vi "Async Cleanup.vi"(8 "error in (no error)":errorcluster, 11 "Variables":T1={"Process Ref"=refnum, "Comm Ref"=refnum, "Bus Info"={"Name"="", "Overrides?"=FALSE, "XNET Refs"={"Incoming"="", "Outgoing"=""}, "Port Info"={"Port"="", "Baud Rate"=0, "Termination"=0, "CAN I/O Mode"=0, "FD Baud Rate"=500000, "Priority"=100, "FD ISO Mode"=0}, "Frames"=variant(cluster{"Convert Session":refnum<k21>, "ID":u32, "Length":i32, "Offset":i32}[] [])}, "Stream Refs"={"Addon"="", "Port"="", "Filter Ref"=refnum, "Default Filter"={"ID Filters"=[], "Direction Filter"=enum."Tx/Rx", "Type Filter"=enum."All"}, "Port Settings"={"Mode"=0, "Baud Rate"=0, "Termination"=0, "FD ISO Mode"=0, "FD Baud Rate"=0}}, "Data Refs"={"Port.Status"=refnum, "Frame.Enable"=refnum, "Frame.Signals"=refnum, "Frame.Overrides"=refnum, "Port.Enable"=refnum}} {"Stream Refs"."Port Settings"."FD ISO Mode" items=["ISO", "Non ISO", "ISO Legacy"]; "Stream Refs"."Port Settings"."Termination" items=["Off", "On"]; "Stream Refs"."Port Settings"."Mode" items=["CAN 2.0", "CAN FD", "CAN FD+BRS"]; "Bus Info"."Port Info"."FD ISO Mode" items=["ISO", "Non ISO", "ISO Legacy"]; "Bus Info"."Port Info"."CAN I/O Mode" items=["CAN 2.0", "CAN FD", "CAN FD+BRS"]; "Bus Info"."Port Info"."Termination" items=["Off", "On"]}) -> (0 "error out":errorcluster)   [LabVIEW 2019, in "Ghost Bus Addon Engine.lvlib"]
uses:
  Ghost Bus Addon Engine.lvlib
  Types/RT Async Engine Variables.ctl
  <vilib>/NI/NIVS Inline Async API/_VS Inline Async API/Process/Process.lvclass
  <vilib>/NI/NI VeriStand Addon Network Comm/Engine/VeriStand Comm.lvclass
  Types/RT Bus Settings.ctl
  Types/RT XNET Refs.ctl
  Addon Shared/Types/XNET Port Settings.ctl
  SubModules/CAN-Streaming-Support/Source/Addon/Addon Engine/Types/Engine Stream Refs.ctl
  SubModules/CAN-Streaming-Support/Source/Addon/Addon Shared/Types/Direction Filter.ctl
  SubModules/CAN-Streaming-Support/Source/Addon/Addon Shared/Types/Type Filter.ctl
  SubModules/CAN-Streaming-Support/Source/Addon/Addon Shared/Types/Filter Parameters.ctl
  SubModules/CAN-Streaming-Support/Source/Addon/Addon Engine/Types/Engine Stream Port Settings.ctl
  Types/RT Data Refs.ctl
  <vilib>/NI/NIVS Inline Async API/_Data Access Engine/Data Access Engine/Types/Write.DVR.ctl
  <vilib>/NI/NIVS Inline Async API/_Data Access Engine/Access Type Classes/Write/Write.lvclass
  <vilib>/NI/NIVS Inline Async API/_Data Access Engine/Data Access Engine/Types/Read.DVR.ctl
  <vilib>/NI/NIVS Inline Async API/_Data Access Engine/Access Type Classes/Read/Read.lvclass
  Types/RT Frame Settings.ctl
  <vilib>/Utility/SystemLogging/Write to System Log.vi
  SubModules/CAN-Streaming-Support/Source/Addon/Addon Shared/CAN Stream Support Shared.lvlib
  SubModules/CAN-Streaming-Support/Source/Addon/Addon Engine/CAN Stream Support Engine.lvlib
  <vilib>/NI/NIVS Inline Async API/_Data Access Engine/Data Access Engine/Data Access Engine.lvclass
  Addon Shared/Ghost Bus Addon Shared.lvlib
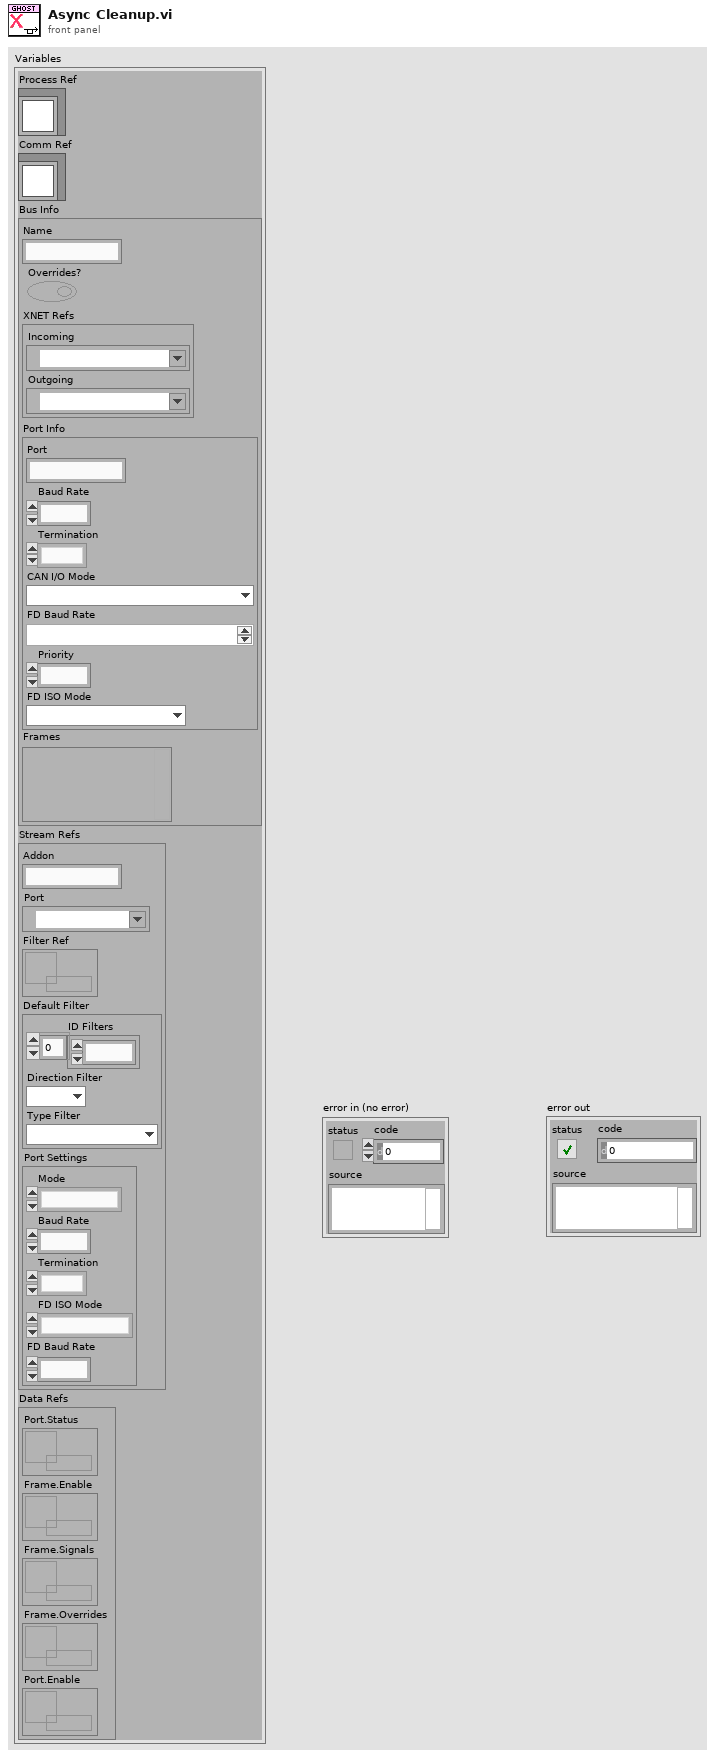
[diagram p1: front panel]
types:
  T1 = typedef "Ghost Bus Addon Engine.lvlib/RT Async Engine Variables.ctl" = cluster{"Process Ref":refnum<class "Process.lvclass">, "Comm Ref":refnum<class "VeriStand Comm.lvclass">, "Bus Info":T2, "Stream Refs":T5, "Data Refs":T10}
  T2 = typedef "RT Bus Settings.ctl" = cluster{"Name":string, "Overrides?":bool, "XNET Refs":T3, "Port Info":T4, "Frames":variant}
  T3 = typedef "Ghost Bus Addon Engine.lvlib/RT XNET Refs.ctl" = cluster{"Incoming":refnum<k21>, "Outgoing":refnum<k21>}
  T4 = typedef "Ghost Bus Addon Shared.lvlib/XNET Port Settings.ctl" = cluster{"Port":string, "Baud Rate":u64, "Termination":u32, "CAN I/O Mode":u32, "FD Baud Rate":u64, "Priority":i32, "FD ISO Mode":u32}
  T5 = typedef "CAN Stream Support Engine.lvlib/Engine Stream Refs.ctl" = cluster{"Addon":string, "Port":refnum<k21>, "Filter Ref":refnum<data-value>, "Default Filter":T6, "Port Settings":T9}
  T6 = typedef "CAN Stream Support Shared.lvlib/Filter Parameters.ctl" = cluster{"ID Filters":u32[], "Direction Filter":T7, "Type Filter":T8}
  T7 = typedef "CAN Stream Support Shared.lvlib/Direction Filter.ctl" = enum16{"Tx/Rx", "Rx", "Tx"}
  T8 = typedef "CAN Stream Support Shared.lvlib/Type Filter.ctl" = enum16{"All", "CAN Data", "CAN Remote", "CAN Bus Error", "CAN 2.0 Data", "CAN FD Data", "CAN FD+BRS Data", "J1939 Data", "Delay", "Log Trigger", "Start Trigger"}
  T9 = typedef "CAN Stream Support Engine.lvlib/Engine Stream Port Settings.ctl" = cluster{"Mode":u32, "Baud Rate":u64, "Termination":u32, "FD ISO Mode":u32, "FD Baud Rate":u64}
  T10 = typedef "Ghost Bus Addon Engine.lvlib/RT Data Refs.ctl" = cluster{"Port.Status":T11, "Frame.Enable":T12, "Frame.Signals":T12, "Frame.Overrides":T12, "Port.Enable":T12}
  T11 = typedef "Data Access Engine.lvlib/Data Access Engine.lvclass/Write.DVR.ctl" = refnum<data-value>
  T12 = typedef "Data Access Engine.lvlib/Data Access Engine.lvclass/Read.DVR.ctl" = refnum<data-value>
  T13 = typedef "Ghost Bus Addon Engine.lvlib/RT Frame Settings.ctl" = cluster{"Convert Session":refnum<k21>, "Length":i32, "Offset":i32, "Enable Offset":i32}
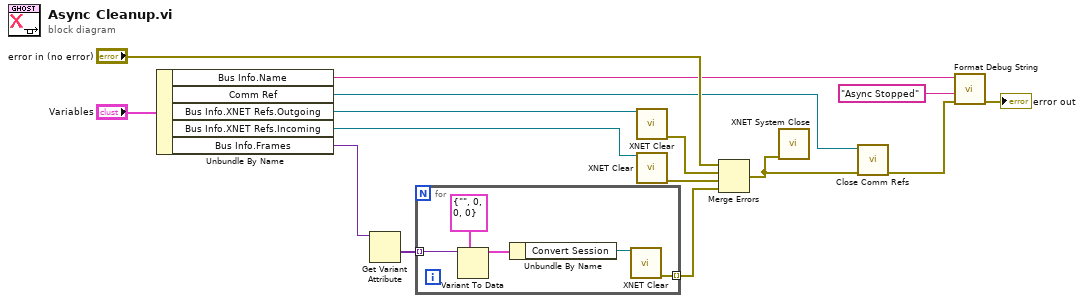
[diagram p0: block diagram]
diagram:
  n1 = Unbundle By Name("Variables") -> ("Bus Info.Name"=w8:string, "Comm Ref"=w3:refnum<class "VeriStand Comm.lvclass">, "Bus Info.XNET Refs.Outgoing"=w15:refnum<k21>, "Bus Info.XNET Refs.Incoming"=w6:refnum<k21>, "Bus Info.Frames"=w2:variant)
  n2 = Get Variant Attribute(Variant=w2) -> (values=w1:variant[])  [unwired: 3 in, 3 out]
  n3 = for {
    tunnel: [w19] -> w4 mode=indexing
    tunnel: w1 -> [w18] mode=indexing
    n4 = Variant To Data(type=T13 {"Convert Session"="", "Length"=0, "Offset"=0, "Enable Offset"=0} ("cluster"), Variant=w18) -> (data=w16:T13)  [unwired: 1 in, 1 out]
    n5 = Unbundle By Name(w16) -> ("Convert Session"=w20:refnum<k21>)
    n6 = call <vilib>:"XNET Clear.vi"("session in"=w20) -> ("error out"=w19:errorcluster)  [unwired: 14 in]
  }
  n7 = call <vilib>:"XNET Clear.vi"("session in"=w15) -> ("error out"=w14:errorcluster)  [unwired: 14 in]
  n8 = call <vilib>:"XNET Clear.vi"("session in"=w6) -> ("error out"=w5:errorcluster)  [unwired: 14 in]
  n9 = Merge Errors("error in (no error)", w14, w5, w4) -> (w11:errorcluster)
  n10 = call <vilib>:"XNET System Close.vi"("error in (no error)"=w11) -> ()  [unwired: 14 in, 1 out]
  n11 = call <vilib>:"Close Comm Refs.vi"("error in"=w11, "Comm.lvclass"=w3) -> ("error out"=w9:errorcluster)  [unwired: 9 in]
  n12 = call "Format Debug String.vi"("error in (no error)"=w9, "State"="Async Stopped", "Name"=w8) -> ("error out"=→"error out":errorcluster)  [unwired: 8 in]
